vi "DB Tools Open Connec (String).vi"(4 "password":string, 5 "userID":string, 6 "error in (no error)":errorcluster, 7 "connection timeout (15)":i32=15, 8 "prompt? (F)":bool, 9 "connection information":string) -> (0 "error out":errorcluster, 3 "connection reference":T2)   [LabVIEW 2013, in "NI_Database_API_64.lvlib"]
doc: "Opens a database connection using the connection information path and returns a connection reference. If <B>prompt?</B> is set to TRUE, LabVIEW displays a dialog box to set up the connection. Wire data to the <B>connection information</B> input to determine the polymorphic instance to use or manually select the instance."
uses:
  NI_Database_API_64.lvlib
  Conn ObjectReference.ctl
  Conn DataMembers.ctl
panel:
  in  "default data":T1
  in  "MSDASC.IDataSourceLocator":refnum<k7>
  in  "ADODB._Connection":refnum<k7>
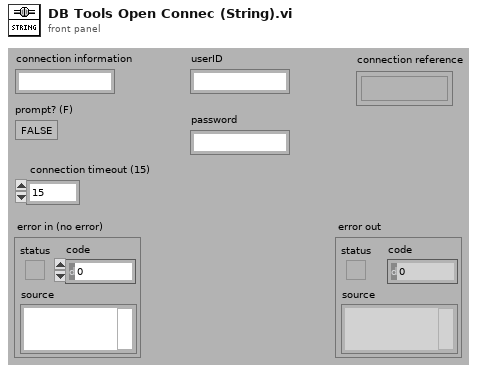
[diagram p1: front panel]
types:
  T1 = typedef "NI_Database_API_64.lvlib/Conn DataMembers.ctl" = cluster{"ADODB._Connection":refnum<k7>, "recordset objects":i32, "command objects":i32}
  T2 = typedef "NI_Database_API_64.lvlib/Conn ObjectReference.ctl" = refnum<k1>
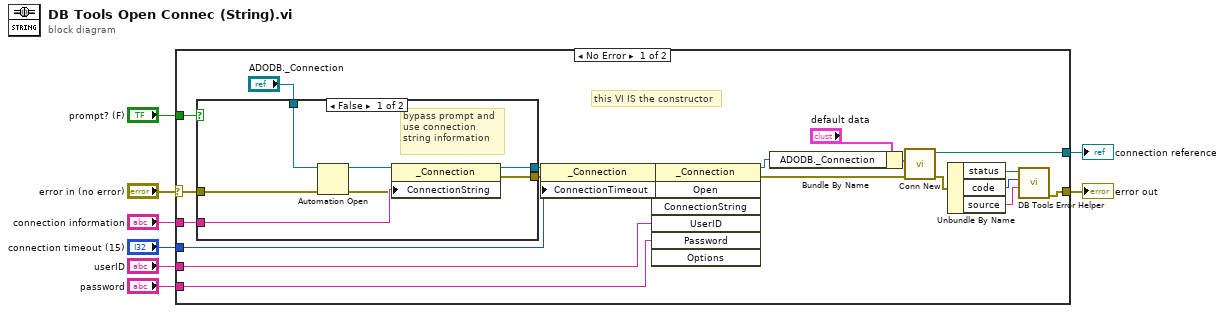
[diagram p0: block diagram]
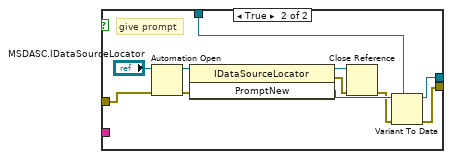
[diagram p2: hidden frame]
diagram:
  n1 = case shown="No Error" "error in (no error)" {
    selector: "error in (no error)" -> [w10 w48]
    tunnel: "userID" -> [w26 _]
    tunnel: "password" -> [w25 _]
    tunnel: "prompt? (F)" -> [w24 _]
    tunnel: [w19 _] -> w5
    tunnel: "connection timeout (15)" -> [w18 _]
    tunnel: [w12 w48] -> w3
    tunnel: "connection information" -> [w11 _]
    frame No Error {
      # "this VI IS the constructor"
      n2 = case shown="False" w24 {
        tunnel: [w36 w41] -> w29
        tunnel: [w35 w42] -> w28
        tunnel: w10 -> [w32 w37]
        tunnel: "ADODB._Connection" -> [w33 w44]
        tunnel: w11 -> [w34 _]
        frame False {
          # "bypass prompt and\nuse connection\nstring information"
          n3 = Automation Open(error in (no error)=w32, Automation Refnum=w33) -> (Automation Refnum=w31:refnum<k7>, error out=w30:errorcluster)  [unwired: 2 out]
          n4 = property class="_Connection"(reference=w31, error in=w30, "ConnectionString"=w34) -> (reference out=w36:refnum<k7>, error out=w35:errorcluster)
        }
        frame True {
          # "give prompt"
          n5 = Automation Open(error in (no error)=w37, Automation Refnum="MSDASC.IDataSourceLocator") -> (Automation Refnum=w38:refnum<k7>, error out=w40:errorcluster)  [unwired: 2 out]
          n6 = invoke class="IDataSourceLocator" method="PromptNew"(reference=w38, error in=w40) -> (reference out=w47:refnum<k7>, error out=w46:errorcluster, "PromptNew"=w45:variant)  [unwired: 1 in]
          n7 = Close Reference(reference=w47, error in (no error)=w46) -> (error out=w43:errorcluster)
          n8 = Variant To Data(error in=w43, type=w44, Variant=w45) -> (data=w41:refnum<k7>, error out=w42:errorcluster)
        }
      }
      n9 = property class="_Connection"(reference=w29, error in=w28, "ConnectionTimeout"=w18) -> (reference out=w22:refnum<k7>, error out=w27:errorcluster)
      n10 = invoke class="_Connection" method="Open"(reference=w22, error in=w27, "UserID"=w26, "Password"=w25) -> (reference out=w9:refnum<k7>, error out=w17:errorcluster)  [unwired: 3 in, 5 out]
      n11 = Bundle By Name(cluster="default data", "ADODB._Connection"=w9) -> (w21:T1)
      n12 = call "Conn New.vi"("error in (no error)"=w17, "initial data"=w21) -> ("error out"=w16:errorcluster, "connection reference"=w19:T2)  [unwired: 4 out]
      n13 = Unbundle By Name(w16) -> ("status"=w15:bool, "code"=w14:i32, "source"=w13:string)
      n14 = call "DB Tools Error Helper.vi"("source"=w13, "code"=w14, "status"=w15) -> ("error out"=w12:errorcluster)  [unwired: 1 in, 7 out]
    }
    frame Error {
    }
  }
  "error out" <- w3
  "connection reference" <- w5
